vi "SV UFF58 Format ASCII Function (Time Waveform) (1 Ch).vi"(1 "ID lines (1-3)":T3, 2 "data precision (DBL:1)":T4=1 items=["single-precision", "double-precision"], 5 "waveform":waveform(dbl)={"t0"=timestamp(0 s since 1904-01-01), "dt"=0.0, "Y"=[]}, 11 "error in (no error)":errorcluster, 12 "DOF Identification":T2 {"response direction" items=["-Z Rotation"=-6, "-Y Rotation"=-5, "-X Rotation"=-4, "-Z Translation"=-3, "-Y Translation"=-2, "-X Translation"=-1, "Scalar"=0, "+X Translation"=1, "+Y Translation"=2, "+Z Translation"=3, "+X Rotation"=4, "+Y Rotation"=5, "+Z Rotation"=6]}) -> (6 "UFF58 ASCII function string":string, 15 "error out":errorcluster)   [LabVIEW 2017, in "SoundVib_UFF58.lvlib"]
doc: "Formats data to the UFF58 (universal file format) ASCII format. This VI also writes the fields in records 1, 2, and 3, <B>ID lines (1-3)</B> as well as all the records and fields associated with the specified instance and the attributes of input data. You can write a single time domain waveform, a single real frequency spectrum, or a complex frequency spectrum to a UFF58 formatted string. If a frequency spectrum is in decibels, this VI converts the spectrum to linear before writing the data to the formatted string. The default instance, SV UFF58 Format ASCII Function (Time Waveform), writes a single time domain waveform to the file specified by the <B>waveform</B> input. Wire data to the <B>waveform</B> input to determine the polymorphic instance to use or manually select the instance."
uses:
  <vilib>/addons/Sound and Vibration/svt_UFF58/SoundVib_UFF58.lvlib
  <vilib>/addons/Sound and Vibration/svt_UFF58/subVIs/sv_UFF58 Data Precision.ctl
  <vilib>/addons/Sound and Vibration/svt_UFF58/subVIs/sv_IDLines123.ctl
  <vilib>/addons/Sound and Vibration/svt_UFF58/subVIs/sv_UFF58 Response Direction.ctl
  <vilib>/addons/Sound and Vibration/svt_UFF58/subVIs/sv_FunctionType.ctl
  <vilib>/addons/Sound and Vibration/svt_UFF58/subVIs/sv_UFF58 Check Data Valid (Time) (1Ch).vi
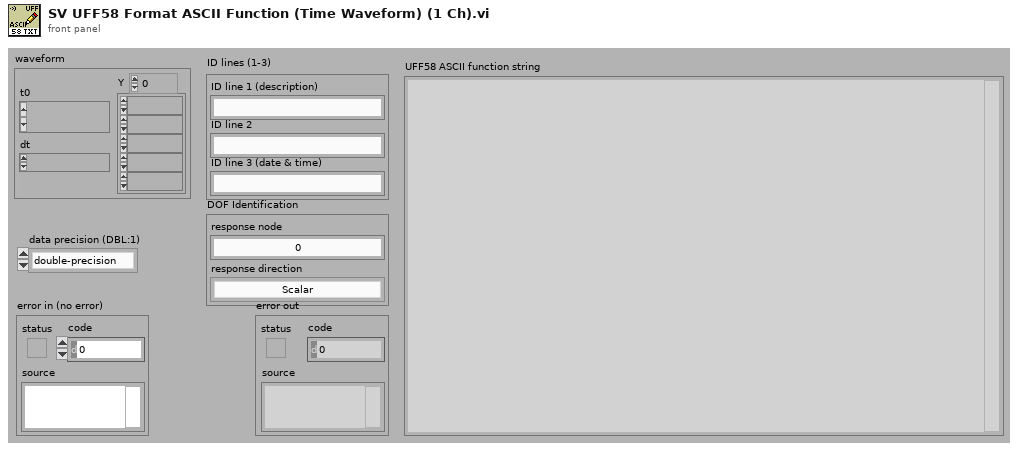
[diagram p1: front panel]
types:
  T1 = typedef "SoundVib_UFF58.lvlib/sv_UFF58 Response Direction.ctl" = i32
  T2 = cluster{"response node":i32, "response direction":T1}
  T3 = typedef "SoundVib_UFF58.lvlib/sv_IDLines123.ctl" = cluster{"ID line 1 (description)":string, "ID line 2":string, "ID line 3 (date & time)":string}
  T4 = typedef "SoundVib_UFF58.lvlib/sv_UFF58 Data Precision.ctl" = u32
  T5 = cluster{"ID line 1":string, "ID line 2":string, "ID line 3":string, "ID line 4":string, "ID line 5":string}
  T6 = cluster{"ordinate data type":u16, "number of data values/pairs":i32, "abscissa spacing":enum16{"uneven", "even"}, "abscissa minimum":dbl, "abscissa increment":dbl, "z-axis value":dbl}
  T7 = typedef "SoundVib_UFF58.lvlib/sv_FunctionType.ctl" = enum16{"general or unknown", "time response", "auto spectrum", "cross spectrum", "frequency response function", "transmissibility", "coherence", "auto correlation", "cross correlation", "power spectral density (PSD)", "energy spectral density (ESD)", "probability density function", "spectrum", "cumulative frequency distribution", "peaks valley", "stress/cycles", "strain/cycles", "orbit", "mode indicator function", "force pattern", "partial power", "partial coherence", "eigenvalue", "eigenvector", "shock response spectrum", "finite impulse response filter", "multiple coherence", "order function", "phase compensation"}
  T8 = typedef "SoundVib_UFF58.lvlib/sv_UFF58 DOF.ctl" = cluster{"function type":T7, "function ID number":i32, "version number":i32, "load case ID number":i32, "response entity name":string, "response node":i32, "response direction":T1, "reference entity name":string, "reference node":i32, "reference direction":T1}
  T9 = typedef "SoundVib_UFF58.lvlib/sv_UFF58 Axis Characteristics.ctl" = cluster{"specific data type":T10, "length units exponent":i32, "force units exponent":i32, "temperature units exponent":i32, "axis label":string, "axis units label":string}
  T10 = typedef "SoundVib_UFF58.lvlib/sv_UFF58 Specific Datatype.ctl" = u16
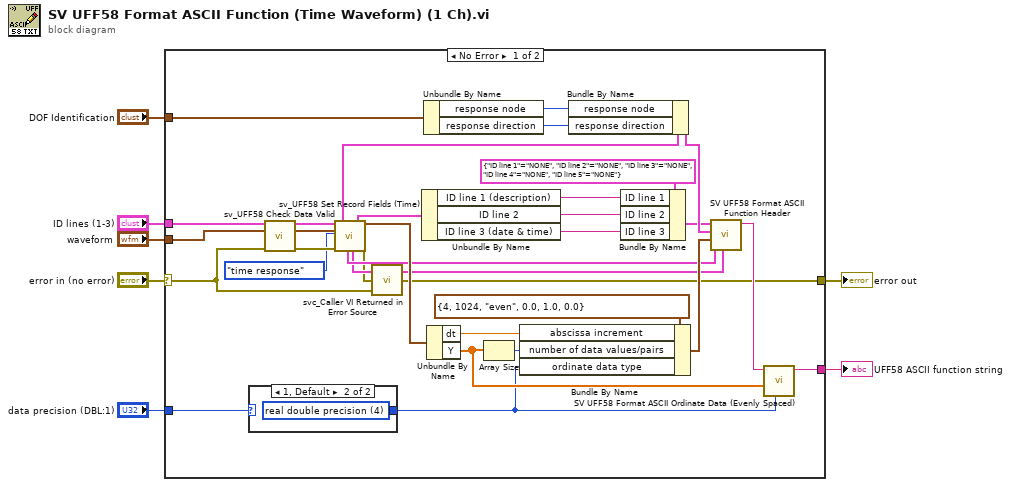
[diagram p0: block diagram]
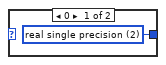
[diagram p2: hidden frame]
diagram:
  n1 = case shown="No Error" "error in (no error)" {
    selector: "error in (no error)" -> [w10 w41]
    tunnel: "data precision (DBL:1)" -> [w12 _]
    tunnel: [w36 _] -> w6
    tunnel: "waveform" -> [w35 _]
    tunnel: "ID lines (1-3)" -> [w22 _]
    tunnel: "DOF Identification" -> [w34 _]
    tunnel: [w8 w41] -> w2
    frame No Error {
      n2 = case shown="1, Default" w12 {
        tunnel: [w39 w40] -> w11
        frame 0 {
          w39 = u16 2 items=["real single precision"=2, "real double precision"=4, "complex single precision"=5, "complex double precision"=6] ("ordinate data type")
        }
        frame 1, Default {
          w40 = u16 4 items=["real single precision"=2, "real double precision"=4, "complex single precision"=5, "complex double precision"=6] ("ordinate data type")
        }
      }
      n3 = call-poly <vilib>:"sv_UFF58 Check Data Valid.vi"("waveform"=w35, "error in (no error)"=w10) -> ("dup waveform"=w20:waveform(dbl), "error out"=w21:errorcluster)  [unwired: 12 in]
      n4 = call <vilib>:"sv_UFF58 Set Record Fields (Time).vi"("ID lines (1-3)"=w22, "waveform"=w20, "function type"=sv_FunctionType."time response", "error in (no error)"=w21) -> ("DOF identification (record 6)"=w14:T8, "abscissa data characteristics (record 8)"=w17:T9, "ordinate numerator data characteristics (record 9)"=w16:T9, "ID lines (1-3) out"=w15:T3, "dup waveform"=w19:waveform(dbl), "error out"=w9:errorcluster)  [unwired: 10 in]
      n5 = call <vilib>:"svc_Caller VI Returned in Error Source.vi"("warning input to caller"=w10, "error in (no error)"=w9) -> ("error out"=w8:errorcluster)  [unwired: 3 in]
      n6 = Unbundle By Name(w15) -> ("ID line 1 (description)"=w29:string, "ID line 2"=w28:string, "ID line 3 (date & time)"=w27:string)
      n7 = Unbundle By Name(w34) -> ("response node"=w33:i32, "response direction"=w32:T1)
      n8 = Unbundle By Name(w19) -> ("dt"=w23:dbl, "Y"=w24:dbl[])
      n9 = Array Size(array=w24) -> (size(s)=w26:i32)
      n10 = Bundle By Name(cluster=T6 {"ordinate data type"=4, "number of data values/pairs"=1024, "abscissa spacing"=enum."even", "abscissa minimum"=0.0, "abscissa increment"=1.0, "z-axis value"=0.0} ("record 7 - data form"), "abscissa increment"=w23, "number of data values/pairs"=w26, "ordinate data type"=w11) -> (w31:T6)
      n11 = Bundle By Name(cluster=w14, "response node"=w33, "response direction"=w32) -> (w25:T8)
      n12 = Bundle By Name(cluster=T5 {"ID line 1"="NONE", "ID line 2"="NONE", "ID line 3"="NONE", "ID line 4"="NONE", "ID line 5"="NONE"} ("ID Lines 1-5"), "ID line 1"=w29, "ID line 2"=w28, "ID line 3"=w27) -> (w13:T5)
      n13 = call <vilib>:"SV UFF58 Format ASCII Function Header.vi"("record 9 - ordinate data characteristics"=w16, "record 8 - abscissa data characteristics"=w17, "record 7 - data form"=w31, "record 6 - DOF identification"=w25, "records (1-5)"=w13) -> ("formatted UFF58 ASCII header"=w38:string)  [unwired: 6 in]
      n14 = call <vilib>:"SV UFF58 Format ASCII Ordinate Data (Evenly Spaced).vi"("ordinate data type"=w11, "ordinate values (Y Re)"=w24, "formatted UFF58 ASCII header"=w38) -> ("UFF58 ASCII function string"=w36:string)  [unwired: 8 in]
    }
    frame Error {
    }
  }
  "UFF58 ASCII function string" <- w6
  "error out" <- w2
